vi "量程参数读取.vi"(8 "error in (no error)":errorcluster caption="错误输入（无错误）", 11 "测量参数":u16(ring) items=["COD"=22, "氨氮"=3, "总氮"=2, "总磷"=1]) -> (0 "error out":errorcluster caption="错误输出", 3 "量程参数读取":T1)   [LabVIEW 2022 SP3, in "斯坦道通用流路CODmn.lvlib"]
uses:
  <vilib>/Plasmionique/MB Master/MB Master.lvlib
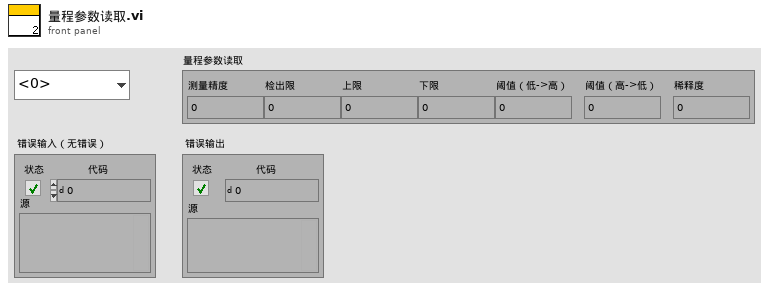
[diagram p1: front panel]
types:
  T1 = cluster{"测量精度":u16, "检出限":dbl, "上限":dbl, "下限":dbl, "阈值（低->高）":dbl, "阈值（高->低）":dbl, "稀释度":dbl}
  T2 = cluster{"FLOAT[0]":sgl, "FLOAT[1]":sgl, "FLOAT[2]":sgl, "FLOAT[3]":sgl, "FLOAT[4]":sgl}
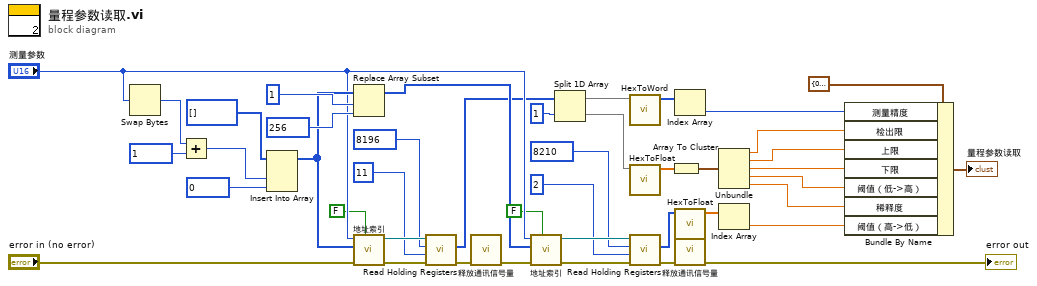
[diagram p0: block diagram]
diagram:
  n1 = Swap Bytes(anything="测量参数") -> (byte swapped=w21:u16)
  n2 = Add(x=w21, y=u16 1 ("starting address")) -> (x+y=w42:u16)
  n3 = Insert Into Array(array=u16[] [] ("数组"), new element #1=w42, new element #2=u16 0 ("starting address")) -> (w15:u16[])  [unwired: 1 in]
  n4 = Replace Array Subset(array=w15, new element=u16 256 ("starting address"), index=1 ("索引")) -> (w10:u16[])
  n5 = call "地址索引.vi"("4.2写公式？"=FALSE ("写流程？"), "error in (no error)"="error in (no error)", "values"=w15, "测量参数"="测量参数") -> ("error out"=w20:errorcluster, "MB session out"=w14:refnum<class "MB_Master.lvclass">)  [unwired: 6 in]
  n6 = call <vilib>:"Read Holding Registers.vi"("error in (no error)"=w20, "quantity"=u16 11, "starting address"=u16 8196, "MB session in"=w14) -> ("error out"=w19:errorcluster, "Registers"=w6:u16[])  [unwired: 5 in, 1 out]
  n7 = call "释放通讯信号量.vi"("error in (no error)"=w19) -> ("error out"=w16:errorcluster)  [unwired: 10 in]
  n8 = call "地址索引.vi"("4.2写公式？"=FALSE ("写流程？"), "error in (no error)"=w16, "values"=w10, "测量参数"="测量参数") -> ("error out"=w17:errorcluster, "MB session out"=w9:refnum<class "MB_Master.lvclass">)  [unwired: 6 in]
  n9 = Split 1D Array(array=w6, index=1 ("长度")) -> (first subarray=w28:u16[], second subarray=w27:u16[])
  n10 = call "HexToWord.vi"("数组"=w28) -> ("WORD"=w38:u16[])  [unwired: 10 in]
  n11 = call "HexToFloat.vi"("数组"=w27) -> ("FLOAT"=w43:sgl[])  [unwired: 10 in]
  n12 = call <vilib>:"Read Holding Registers.vi"("error in (no error)"=w17, "quantity"=u16 2, "starting address"=u16 8210, "MB session in"=w9) -> ("error out"=w18:errorcluster, "Registers"=w5:u16[])  [unwired: 5 in, 1 out]
  n13 = Array To Cluster(array=w43) -> (cluster=w36:T2)
  n14 = Index Array(array=w38) -> (element=w37:u16)  [unwired: 1 in]
  n15 = call "HexToFloat.vi"("数组"=w5) -> ("FLOAT"=w30:sgl[])  [unwired: 10 in]
  n16 = call "释放通讯信号量.vi"("error in (no error)"=w18) -> ("error out"=→"error out":errorcluster)  [unwired: 10 in]
  n17 = Unbundle(w36) -> ("FLOAT[0]"=w35:sgl, "FLOAT[1]"=w34:sgl, "FLOAT[2]"=w33:sgl, "FLOAT[3]"=w32:sgl, "FLOAT[4]"=w31:sgl)
  n18 = Index Array(array=w30) -> (element=w24:sgl)  [unwired: 1 in]
  n19 = Bundle By Name(cluster=T1 {"测量精度"=0, "检出限"=0.0, "上限"=0.0, "下限"=0.0, "阈值（低->高）"=0.0, "阈值（高->低）"=0.0, "稀释度"=0.0} ("量程参数读取"), "测量精度"=w37, "检出限"=w35, "上限"=w34, "下限"=w33, "阈值（低->高）"=w32, "稀释度"=w31, "阈值（高->低）"=w24) -> (→"量程参数读取":T1)
